vi "1_ArrayU8_To_Image.vi"(0 "Array Src IN":u8[](array[numeric]), 1 "Buffer Image":T1, 3 "Width":i32, 4 "Height":i32, 5 "Error in":errorcluster caption="Error in (no error)") -> (15 "Image":T1(plugin-control), 19 "Error out":errorcluster={"status"=FALSE, "code"=0, "source"="\n  "})   [LabVIEW 2018]
doc: "It converts a 1D Array U8 to image It receives un 1D Array U8, the buffer that reserve memory for the image and the width and the height of the image."
uses:
  <vilib>/vision/Image Controls.llb/IMAQ Image.ctl
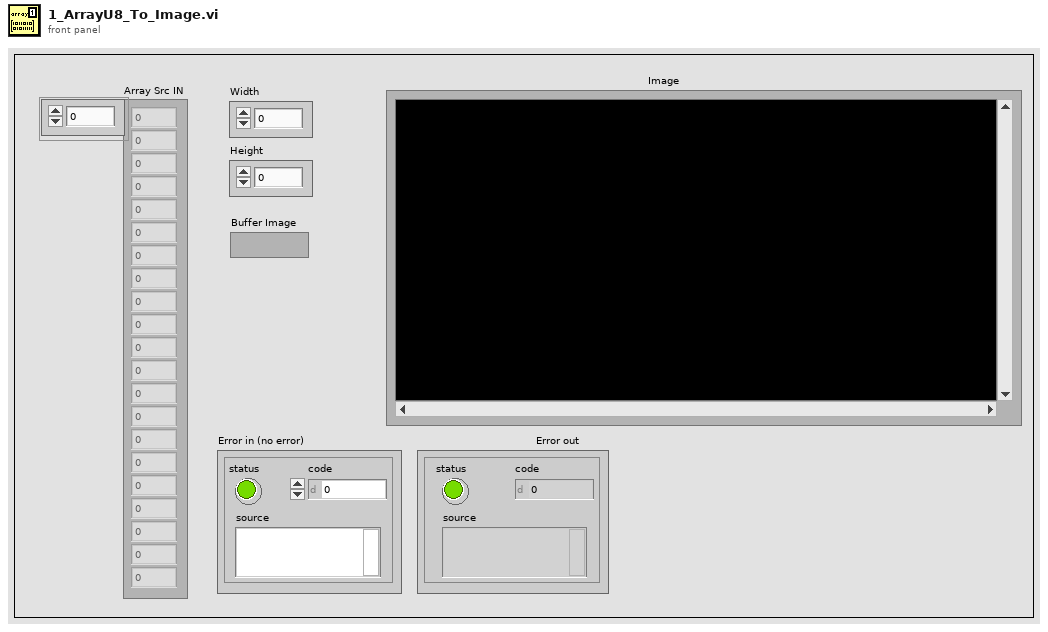
[diagram p1: front panel]
types:
  T1 = typedef "IMAQ Image.ctl" = refnum<image>
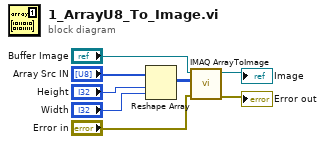
[diagram p0: block diagram]
diagram:
  n1 = Reshape Array("Array Src IN", "Height", "Width") -> (w8:u8[][])
  n2 = call "IMAQ ArrayToImage"("error in (no error)"="Error in", "Image Pixels (U8)"=w8, "Image"="Buffer Image") -> ("error out"=→"Error out":errorcluster, "Image Out"=→"Image":T1)  [unwired: 7 in]
